vi "LSM9DS1_MagSetup.vi"(8 "error in (no error)":errorcluster, 10 "Mag_Settings":T1={"Mag_Range"=enum."±2 gauss", "Mag_Address"=enum."0x1E", "Anomaly Thresh"=0.0, "Local Mag"=0.0}, 11 "I2C Bus":T3=enum."Invalid") -> (0 "error out":errorcluster, 2 "Mag_Active":bool, 3 "I2CMagDevRef":T2={"DevStatus"={"status"=FALSE, "code"=0, "source"=""}, "Device Address"=0, "Handle"=0, "I2C Bus"=enum."Invalid"} {"Device Address" format="%.0x"})   [LabVIEW 2015]
uses:
  <vilib>/Rock Robotics/SystemInterfaces/i2clib/i2c_bus.ctl
  <vilib>/Rock Robotics/WPI/I2C/WPI_I2CDevRef.ctl
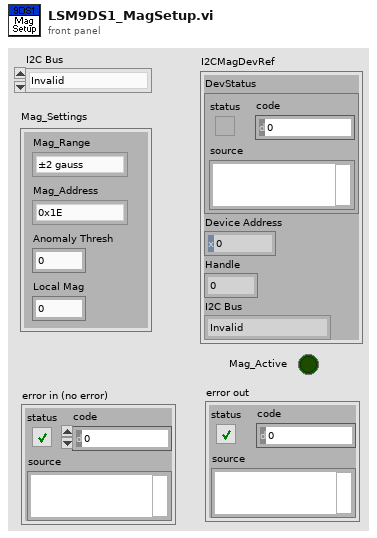
[diagram p1: front panel]
types:
  T1 = cluster{"Mag_Range":enum8{"±2 gauss", "±4 gauss", "±8 gauss", "±16 gauss", "disabled"}, "Mag_Address":enum8{"0x1C", "0x1E"}, "Anomaly Thresh":dbl, "Local Mag":dbl}
  T2 = typedef "WPI_I2CDevRef.ctl" = cluster{"DevStatus":errorcluster, "Device Address":u8, "Handle":i32, "I2C Bus":T3}
  T3 = typedef "i2c_bus.ctl" = enum16{"I2C On-Board", "I2C MXP", "Invalid"}
  T4 = enum8{"±2 gauss", "±4 gauss", "±8 gauss", "±16 gauss", "disabled"}
  T5 = cluster{"I2C Bus":T3, "Mag_Settings":cluster{"Mag_Range":enum8{"±2 gauss", "±4 gauss", "±8 gauss", "±16 gauss", "disabled"}, "Mag_Address":enum8{"0x1C", "0x1E"}, "Anomaly Thresh":dbl, "Local Mag":dbl}}
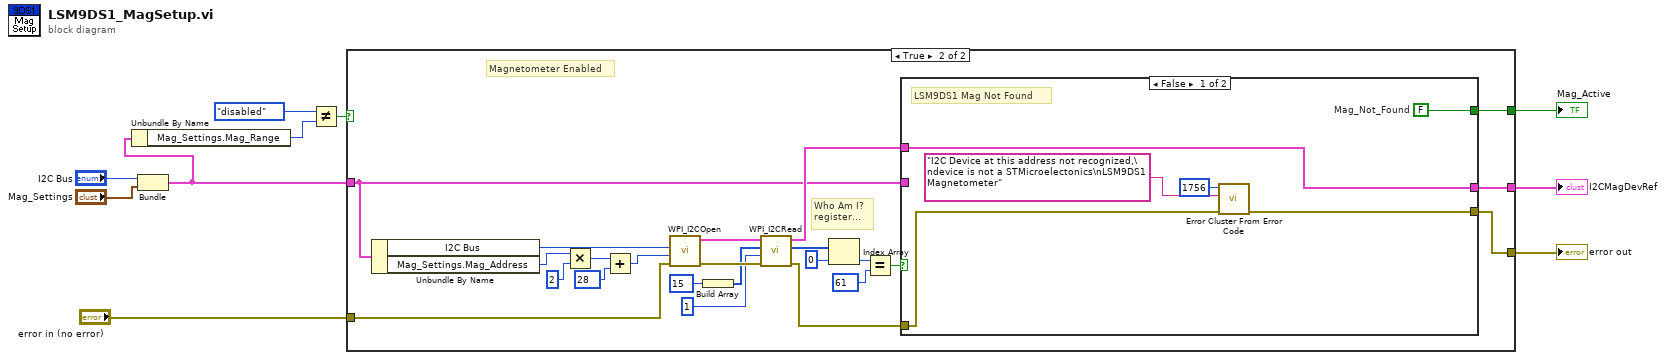
[diagram p0: block diagram]
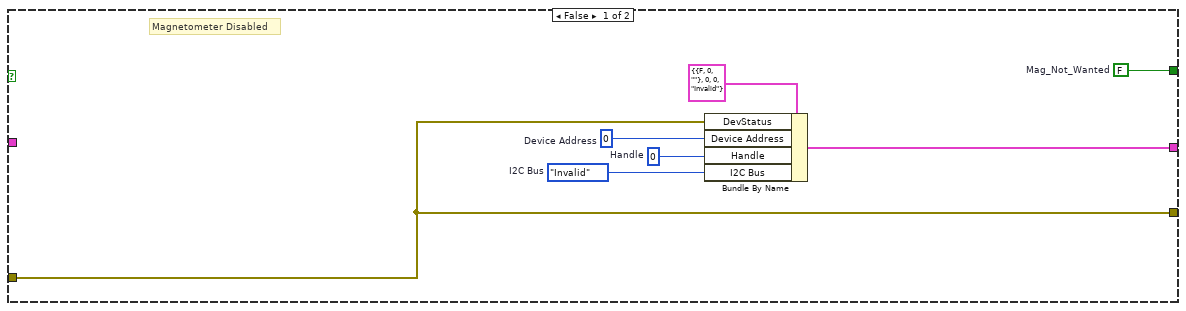
[diagram p2: hidden frame]
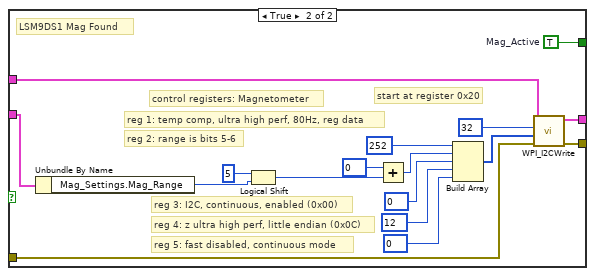
[diagram p3: hidden frame]
diagram:
  n1 = Bundle("I2C Bus"="I2C Bus", "Mag_Settings"="Mag_Settings") -> (w2:T5)  [unwired: 1 in]
  n2 = Unbundle By Name(w2) -> ("Mag_Settings.Mag_Range"=w6:T4)
  n3 = Not Equal?(x=T4."disabled" ("Mag_Settings"), y=w6) -> (x != y?=w7:bool)
  n4 = case shown="True" w7 {
    tunnel: "error in (no error)" -> [w17 w38]
    tunnel: w2 -> [_ w25]
    tunnel: [w17 w26] -> w5
    tunnel: [w12 w24] -> w4
    tunnel: [w11 w18] -> w1
    frame False {
      w11 = FALSE  # Mag_Not_Wanted
      w14 = i2c_bus."Invalid"  # I2C Bus
      w15 = 0  # Handle
      w16 = u8 0  # Device Address
      # "Magnetometer Disabled"
      n5 = Bundle By Name(cluster=T2 {"DevStatus"={"status"=FALSE, "code"=0, "source"=""}, "Device Address"=0, "Handle"=0, "I2C Bus"=enum."Invalid"} ("Array"), "DevStatus"=w17, "Device Address"=w16, "Handle"=w15, "I2C Bus"=w14) -> (w12:T2)
    }
    frame True {
      # "Magnetometer Enabled"
      # "Who Am I?\nregister..."
      n6 = Unbundle By Name(w25) -> ("I2C Bus"=w37:T3, "Mag_Settings.Mag_Address"=w19:enum8{"0x1C", "0x1E"})
      n7 = Multiply(x=w19, y=u8 2) -> (x*y=w23:u8)
      n8 = Add ("Gyro/Accel Slave Address")(x=w23, y=u8 28) -> (x+y=w20:u8)
      n9 = call <vilib>:"WPI_I2COpen.vi"("error in"=w38, "Device Address"=w20, "I2C Bus"=w37) -> ("error out"=w35:errorcluster, "I2CDevRef"=w36:T2)  [unwired: 7 in]
      n10 = Build Array(u8 15 ("I2CRegister")) -> (w33:u8[])
      n11 = call <vilib>:"WPI_I2CRead.vi"("error in (no error)"=w35, "I2CBytesToRead"=u8 1, "I2CRegister"=w33, "I2CDevRef"=w36) -> ("error out"=w27:errorcluster, "Data Out"=w31:u8[], "I2CDevRef"=w29:T2)  [unwired: 5 in]
      n12 = Index Array(array=w31, index=0) -> (element=w39:u8)
      n13 = Equal?(x=w39, y=u8 61) -> (x = y?=w28:bool)
      n14 = case shown="False" w28 {
        tunnel: w29 -> [w42 w53]
        tunnel: w27 -> [w44 w52]
        tunnel: [w43 w51] -> w26
        tunnel: w25 -> [_ w50]
        tunnel: [w42 w48] -> w24
        tunnel: [w41 w47] -> w18
        frame False {
          w41 = FALSE  # Mag_Not_Found
          # "LSM9DS1 Mag Not Found"
          n15 = call <vilib>:"Error Cluster From Error Code.vi"("error in (no error)"=w44, "error message (\"\")"="I2C Device at this address not recognized,\ndevice is not a STMicroelectonics\nLSM9DS1 Magnetometer" ("error message (\"\")"), "error code (0)"=1756) -> ("error out"=w43:errorcluster)  [unwired: 6 in]
        }
        frame True {
          w47 = TRUE  # Mag_Active
          # "reg 5: fast disabled, continuous mode"
          # "reg 1: temp comp, ultra high perf, 80Hz, reg data"
          # "LSM9DS1 Mag Found"
          # "reg 4: z ultra high perf, little endian (0x0C)"
          # "reg 3: I2C, continuous, enabled (0x00)"
          # "reg 2: range is bits 5-6"
          # "start at register 0x20"
          # "control registers: Magnetometer"
          n16 = Unbundle By Name(w50) -> ("Mag_Settings.Mag_Range"=w49:T4)
          n17 = Logical Shift(y=u8 5, x=w49) -> (x << y=w62:u32)
          n18 = Add(x=u8 0, y=w62) -> (x+y=w57:u8)
          n19 = Build Array(u8 252 ("element"), w57, u8 0 ("x"), u8 12 ("element"), u8 0 ("x")) -> (w60:u8[])
          n20 = call <vilib>:"WPI_I2CWrite.vi"("error in (no error)"=w52, "I2CDataToSend"=w60, "I2CRegister"=u8 32 ("element"), "I2CDevRef"=w53) -> ("error out"=w51:errorcluster, "I2CDevRef"=w48:T2)  [unwired: 6 in]
        }
      }
    }
  }
  "error out" <- w5
  "I2CMagDevRef" <- w4
  "Mag_Active" <- w1
